vi "Write limit_alarm_max.vi"(8 "error in (no error)":errorcluster, 10 "limit_alarm_max":dbl, 11 "DAQmxTaskAICurrent_General in":refnum<class "DAQmxTaskAICurrent_General.lvclass">) -> (0 "error out":errorcluster, 3 "DAQmxTaskAICurrent_General out":refnum<class "DAQmxTaskAICurrent_General.lvclass">)   [LabVIEW 2020, in "DAQmxTaskAICurrent_General.lvclass"]
uses:
  DAQmxTaskAICurrent_General.lvclass
  DAQmxTaskAICurrent_General.lvclass/DAQmxTaskAICurrent_General.ctl
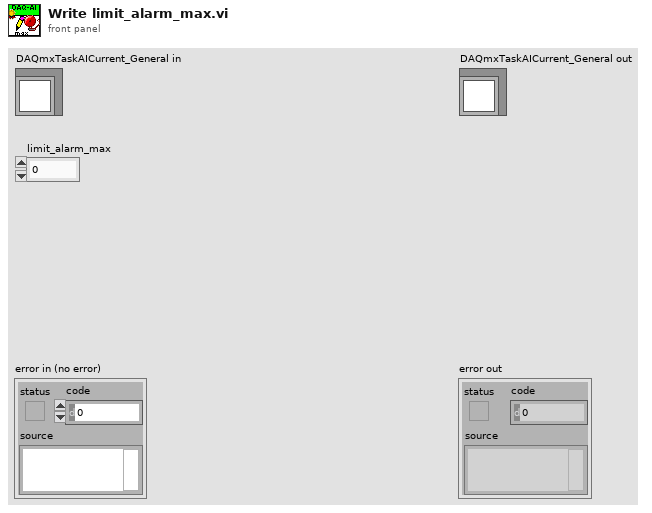
[diagram p1: front panel]
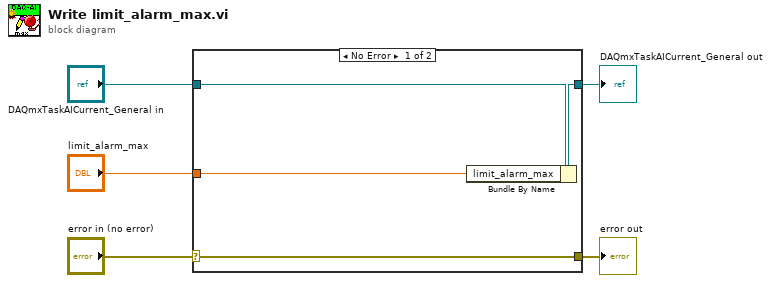
[diagram p0: block diagram]
diagram:
  n1 = case shown="No Error" "error in (no error)" {
    selector: "error in (no error)" -> [w9 w10]
    tunnel: [w9 w10] -> w4
    tunnel: [w7 w11] -> w2
    tunnel: "DAQmxTaskAICurrent_General in" -> [w8 w11]
    tunnel: "limit_alarm_max" -> [w6 _]
    frame No Error {
      n2 = Bundle By Name(cluster=w8, "limit_alarm_max"=w6) -> (w7:refnum<class "DAQmxTaskAICurrent_General.lvclass">)
    }
    frame Error {
    }
  }
  "error out" <- w4
  "DAQmxTaskAICurrent_General out" <- w2
